vi "Calculation chance.vi"(0 "Number of details":i32, 2 "Defective (%)":dbl) -> (1 "Defectives":i32)   [LabVIEW 2020]
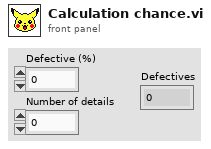
[diagram p1: front panel]
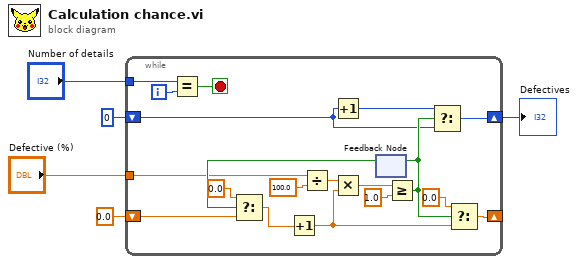
[diagram p0: block diagram]
diagram:
  n1 = while {
    shift-right: [w24] -> _
    shift-left: 0.0 ("t") -> [w21]
    shift-right: [w13] -> w3
    shift-left: 0 -> [w16]
    tunnel: "Defective (%)" -> [w7]
    tunnel: "Number of details" -> [w6]
    i -> [w14]
    stop <- w15 stop-if-true
    n2 = Equal?(x=w6, y=w14) -> (x = y?=w15:bool)
    n3 = Divide(x=w7, y=100.0) -> (x/y=w11:dbl)
    n4 = Increment(x=w16) -> (x+1=w17:i32)
    n5 = feedback #1() -> (w19:bool)  [unwired: 1 in]
    n6 = Select(t=0.0, s=w19, f=w21) -> (s? t:f=w20:dbl)
    n7 = Increment(x=w20) -> (x+1=w8:dbl)
    n8 = Multiply(x=w11, y=w8) -> (x*y=w9:dbl)
    n9 = Greater Or Equal?(x=w9, y=1.0 ("x")) -> (x >= y?=w18:bool)
    n10 = feedback-in #1(w18) -> ()
    n11 = Select(t=w17, s=w18, f=w16) -> (s? t:f=w13:i32)
    n12 = Select(t=0.0, s=w18, f=w8) -> (s? t:f=w24:dbl)
  }
  "Defectives" <- w3
